vi "DDVL Adjust Spacing and Visibility.vi"(0 "Cluster Ref Array":refnum<vi>[](array[refnum]), 2 "Position Index":i32, 11 "Sub Panel Ref Array":refnum<vi>[](array[refnum]), 13 "Num of VIs":i32) -> (15 "Sub Panel Ref Array Dup":refnum<vi>[](array[refnum]))   [LabVIEW 2016]
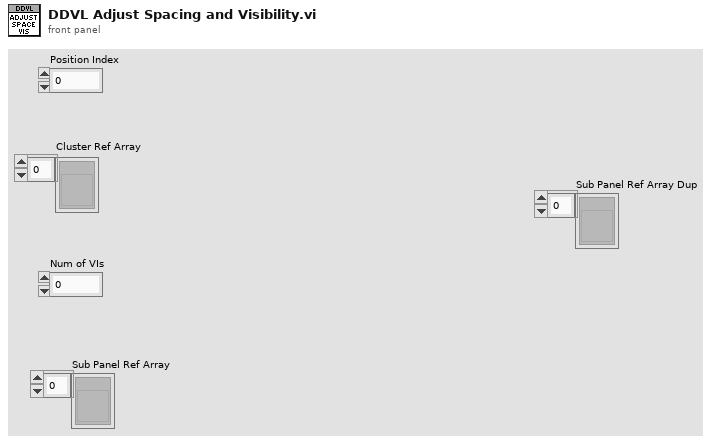
[diagram p1: front panel]
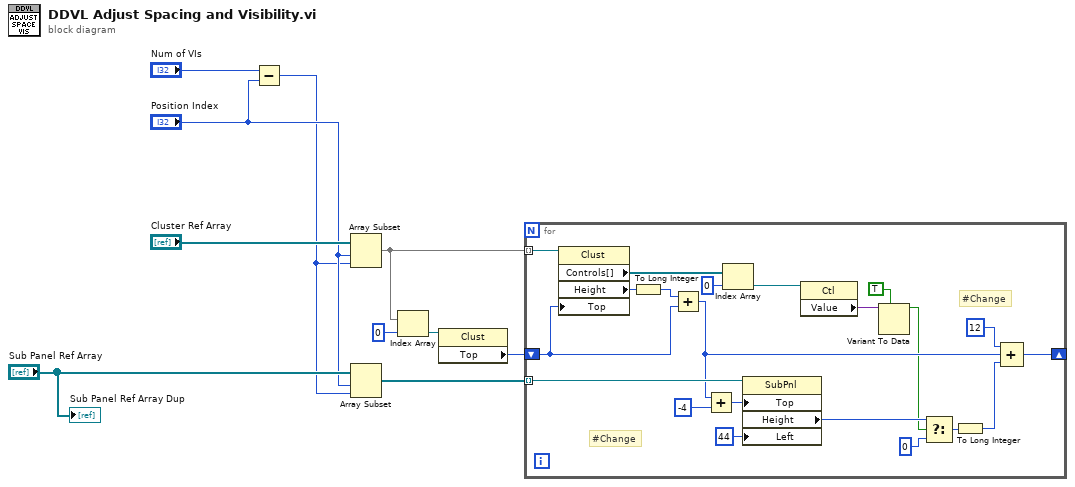
[diagram p0: block diagram]
diagram:
  n1 = Subtract(x="Num of VIs", y="Position Index") -> (x-y=w1:i32)
  n2 = Array Subset(array="Cluster Ref Array", index="Position Index", length=w1) -> (w7:refnum<vi>[])
  n3 = Array Subset(array="Sub Panel Ref Array", index="Position Index", length=w1) -> (w8:refnum<vi>[])
  n4 = Index Array(array=w7, index=0) -> (element=w5:refnum<vi>)
  n5 = property class="Clust"(reference=w5) -> ("Top"=w4:i32)  [unwired: 1 in, 2 out]
  n6 = for {
    tunnel: w7 -> [w31] mode=indexing
    tunnel: w8 -> [w28] mode=indexing
    shift-right: [w22] -> _
    shift-left: w4 -> [w19]
    # "#Change"
    # "#Change"
    n7 = property class="Clust"(reference=w31, "Top"=w19) -> ("Controls[]"=w17:refnum<vi>[], "Height"=w30:u32)  [unwired: 1 in, 2 out]
    n8 = To Long Integer(number=w30) -> (32bit integer=w29:i32)
    n9 = Add(x=w29, y=w19) -> (x+y=w18:i32)
    n10 = Add(x=w18, y=-4) -> (x+y=w26:i32)
    n11 = Index Array(array=w17, index=0) -> (element=w15:refnum<vi>)
    n12 = property class="SubPnl"(reference=w28, "Top"=w26, "Left"=44 ("Position:Left")) -> ("Height"=w25:u32)  [unwired: 1 in, 2 out]
    n13 = property class="Ctl"(reference=w15) -> ("Value"=w14:variant)  [unwired: 1 in, 2 out]
    n14 = Variant To Data(type=TRUE, Variant=w14) -> (data=w12:bool)  [unwired: 1 in, 1 out]
    n15 = Select(t=w25, s=w12, f=u32 0) -> (s? t:f=w23:u32)
    n16 = To Long Integer(number=w23) -> (32bit integer=w20:i32)
    n17 = Compound Arithmetic op=ADD(12 ("x"), w18, w20) -> (w22:i32)
  }
  "Sub Panel Ref Array Dup" <- "Sub Panel Ref Array"
